vi "Query.vi"(5 "buffered":bool=TRUE, 6 "commandTimeout":i32=-1, 7 "CommandType":i32(ring)=-1 items=["Text"=1, "StoredProcedure"=4, "TableDirect"=512], 8 "error in (no error)":errorcluster, 9 "DynamicParameters":refnum<class "DynamicParameters.lvclass">, 10 "sql":string, 11 "SqlMapper in":refnum<class "DapperMapper.lvclass">) -> (0 "error out":errorcluster, 2 "Query Result out":refnum<class "Query Result.lvclass">, 3 "SqlMapper out":refnum<class "DapperMapper.lvclass">)   [LabVIEW 2020, in "ORM_Dapper.lvlib" / "DapperMapper.lvclass"]
uses:
  DapperMapper.lvclass
  C:/Program Files/National Instruments/LabVIEW 2020/vi.lib/Viviota/shared/ORM.lvlibp/ORM/SqlMapper/SqlMapper.lvclass
  <vilib>/Viviota/shared/ORM.lvlibp/ORM/Query Result/Query Result.lvclass
  <vilib>/Viviota/shared/ORM.lvlibp/ORM/DynamicParameters/DynamicParameters.lvclass
  DapperParameters/DapperParameters.lvclass
  <vilib>/Viviota/shared/ORM_DBC_dotNet.lvlibp/dbcDotNet/ORM_DBC_dotNet.lvclass
  DapperParameters/DapperParameters.lvclass/DapperParameters.ctl
  C:/Viviota/Projects/R&D/__OpenSource/VIV_ORM/libraries/dapper/Dapper.dll
  libraries/dapper/Dapper.dll
  DapperResult/DapperResult.lvclass
  C:/Program Files/National Instruments/LabVIEW 2020/vi.lib/Viviota/shared/ORM.lvlibp/ORM/Query Result/Query Result.lvclass
  <vilib>/Viviota/shared/ORM.lvlibp/ORM/SqlMapper/Read DbConnection.vi
  <vilib>/Viviota/shared/ORM_DBC_dotNet.lvlibp/dbcDotNet/Read connection.vi
  <vilib>/Viviota/shared/ORM_DBC_dotNet.lvlibp/dbcDotNet/Read transaction.vi
  <vilib>/Viviota/shared/ORM.lvlibp/ORM/DbConnection/DbConnection.lvclass
  System.Data
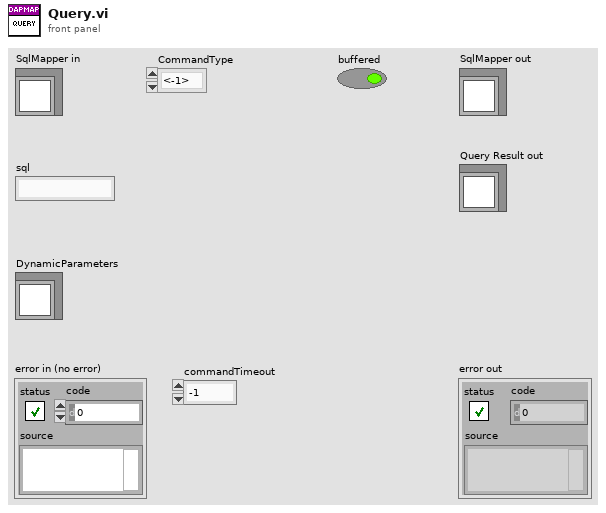
[diagram p1: front panel]
types:
  T1 = typedef "ORM_Dapper.lvlib/dapper_dynamicparameters_ref.ctl" = refnum<k24>
  T2 = typedef "ORM_Dapper.lvlib/dapper_sqlmapper_ref.ctl" = refnum<k24>
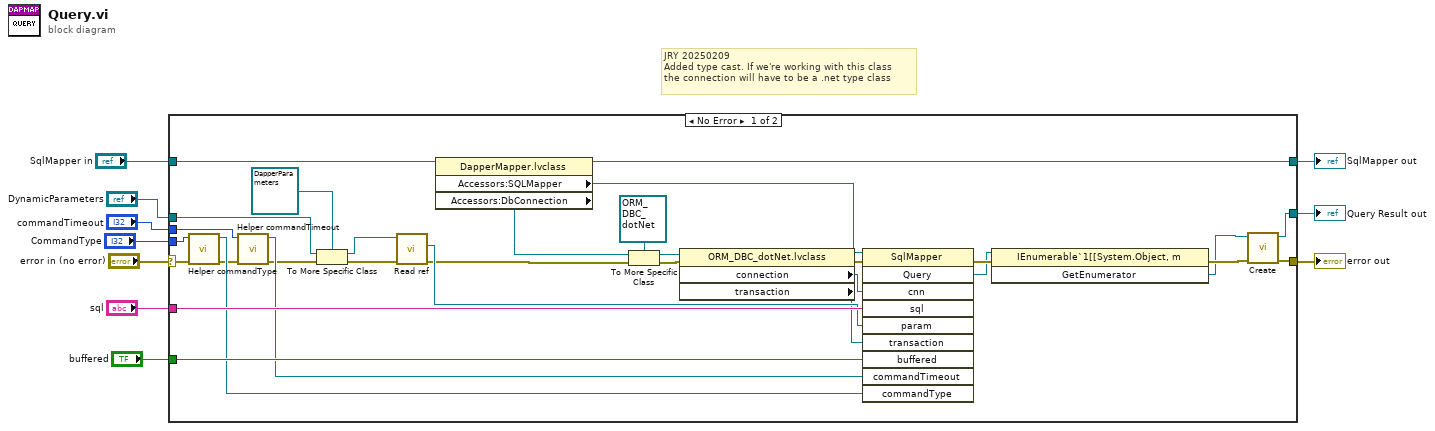
[diagram p0: block diagram]
diagram:
  # "JRY 20250209\nAdded type cast. If we're working with this class\nthe connection will have to be a .net type class"
  n1 = case shown="No Error" "error in (no error)" {
    selector: "error in (no error)" -> [w31 w43]
    tunnel: [w18 w43] -> w9
    tunnel: [w23 w42] -> w7
    tunnel: "SqlMapper in" -> [w30 w42]
    tunnel: "sql" -> [w41 _]
    tunnel: [w15 _] -> w5
    tunnel: "buffered" -> [w38 _]
    tunnel: "CommandType" -> [w36 _]
    tunnel: "commandTimeout" -> [w35 _]
    tunnel: "DynamicParameters" -> [w21 _]
    frame No Error {
      n2 = call "Helper commandType.vi"("error in (no error)"=w31, "CommandType"=w36) -> ("error out"=w32:errorcluster, ".NET Refnum out"=w33:refnum<k24>)  [unwired: 8 in]
      n3 = call "Helper commandTimeout.vi"("error in (no error)"=w32, "commandTimeout in"=w35) -> ("error out"=w29:errorcluster, ".NET Refnum out"=w34:refnum<k24>)  [unwired: 8 in]
      n4 = To More Specific Class(target class=refnum<class "DapperParameters.lvclass"> refnum ("Dapper.lvlib:DynamicParameters"), reference=w21, error in=w29) -> (specific class reference=w20:refnum<class "DapperParameters.lvclass">, error out=w22:errorcluster)
      n5 = call "Read ref.vi"("error in (no error)"=w22, "DynamicParameters in"=w20) -> ("error out"=w25:errorcluster, "ref"=w37:T1)  [unwired: 7 in, 1 out]
      n6 = property class="DapperMapper.lvclass"(reference=w30) -> (reference out=w23:refnum<class "DapperMapper.lvclass">, "Accessors:SQLMapper"=w24:T2, "Accessors:DbConnection"=w13:refnum<class "DbConnection.lvclass">)  [unwired: 1 in, 1 out]
      n7 = To More Specific Class(target class=refnum<class "ORM_DBC_dotNet.lvclass"> refnum ("ORM_DBC_dotNet.lvlibp:ORM_DBC_dotNet.lvclass"), reference=w13, error in=w25) -> (specific class reference=w12:refnum<class "ORM_DBC_dotNet.lvclass">, error out=w14:errorcluster)
      n8 = property class="ORM_DBC_dotNet.lvclass"(reference=w12, error in=w14) -> (error out=w26:errorcluster, "connection"=w28:refnum<k24>, "transaction"=w27:refnum<k24>)  [unwired: 1 out]
      n9 = invoke class="SqlMapper" method="Query"(reference=w24, error in=w26, "cnn"=w28, "sql"=w41, "param"=w37, "transaction"=w27, "buffered"=w38, "commandTimeout"=w34, "commandType"=w33) -> (error out=w40:errorcluster, "Query"=w39:refnum<k24>)  [unwired: 1 in, 8 out]
      n10 = invoke class="IEnumerable`1[[System.Object, m" method="GetEnumerator"(reference=w39, error in=w40) -> (error out=w17:errorcluster, "GetEnumerator"=w16:refnum<k24>)  [unwired: 1 in, 1 out]
      n11 = call "Create.vi"("error in (no error)"=w17, "ref"=w16) -> ("error out"=w18:errorcluster, "Query Result out"=w15:refnum<class "DapperResult.lvclass">)  [unwired: 8 in]
    }
    frame Error {
    }
  }
  "error out" <- w9
  "SqlMapper out" <- w7
  "Query Result out" <- w5
